vi "set_voltage_and_current.vi"(8 "error in 2":errorcluster, 9 "current":dbl, 10 "voltage":dbl, 11 "VISA resource name 2":refnum<visa-resource-name>="COM1") -> (0 "error out 2":errorcluster, 2 "command":string, 3 "VISA resource name out":refnum<visa-resource-name>)   [LabVIEW 2020]
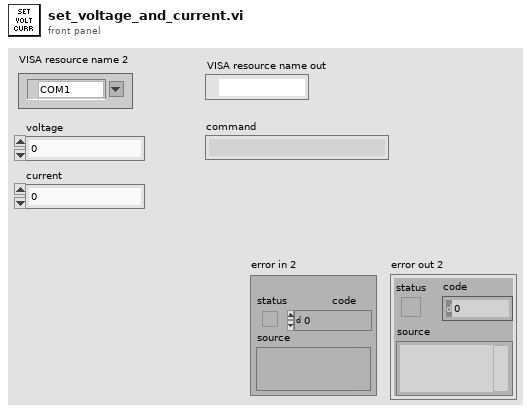
[diagram p1: front panel]
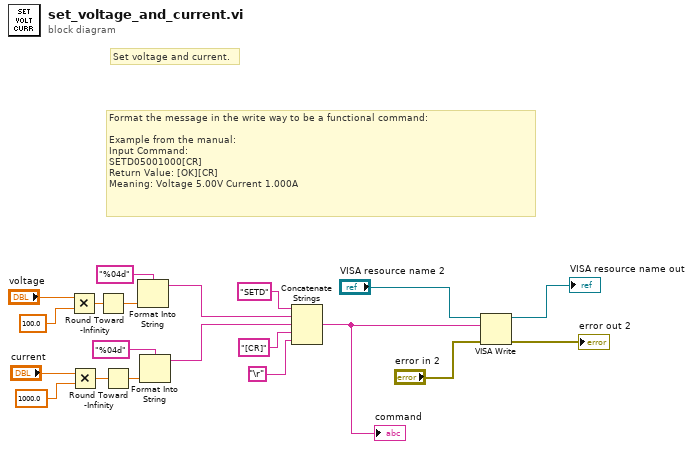
[diagram p0: block diagram]
diagram:
  # "Set voltage and current."
  # "Format the message in the write way to be a functional command:\n\nExample from the manual:\nInput Command:\nSETD05001000[CR]\nReturn Value: [OK][CR]\nMeaning: Voltage 5.00V Current 1.000A"
  n1 = Multiply(x="voltage", y=100.0) -> (x*y=w14:dbl)
  n2 = Multiply(x="current", y=1000.0) -> (x*y=w13:dbl)
  n3 = Round Toward -Infinity(1:w14) -> (0:w10:dbl)
  n4 = Round Toward -Infinity(1:w13) -> (0:w8:dbl)
  n5 = Format Into String(format string="%04d", w10) -> (resulting string=w11:string)  [unwired: 2 in, 1 out]
  n6 = Format Into String(format string="%04d", w8) -> (resulting string=w7:string)  [unwired: 2 in, 1 out]
  n7 = Concatenate Strings("SETD" ("string"), w11, w7, "[CR]" ("string"), "\r") -> (w1:string)
  "command" <- w1
  n8 = VISA Write(VISA resource name="VISA resource name 2", write buffer=w1, error in (no error)="error in 2") -> (VISA resource name out=→"VISA resource name out":refnum<visa-resource-name>, error out=→"error out 2":errorcluster)  [unwired: 1 out]
